vi "Then.vi"(8 "error in (no error)":errorcluster, 9 "Scope":variant, 10 "Callback":refnum<vi>, 11 "Future in":refnum<class "Future.lvclass">) -> (0 "error out":errorcluster)   [LabVIEW 2017, in "Promise Future.lvlib" / "Future.lvclass"]
uses:
  Future.lvclass
  Future.lvclass/Future.ctl
  State/State.lvclass
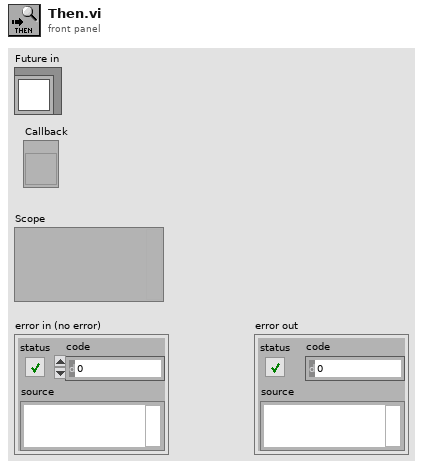
[diagram p1: front panel]
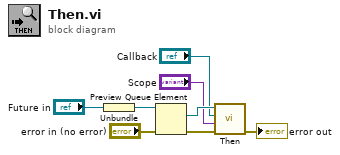
[diagram p0: block diagram]
diagram:
  n1 = Unbundle("Future in") -> (w5:refnum<queue>)
  n2 = Preview Queue Element(queue=w5, error in (no error)="error in (no error)") -> (element=w6:refnum<class "State.lvclass">, error out=w8:errorcluster)  [unwired: 1 in, 2 out]
  n3 = call "Then.vi"("error in (no error)"=w8, "Scope"="Scope", "Callback"="Callback", "State in"=w6) -> ("error out"=→"error out":errorcluster)  [unwired: 7 in]
